vi "set dsf config session.vi"(8 "error in (no error)":errorcluster, 10 "Configuration Session":refnum<class "Configuration Session.lvclass">, 11 "Item Ref in":T1 format="%.0x") -> (0 "error out":errorcluster, 3 "Item Ref out":T1 format="%.0x")   [LabVIEW 2017, in "DSF System Explorer.lvlib"]
uses:
  DSF System Explorer.lvlib
  <vilib>/NI Veristand/Custom Device API/Custom Device Item Ref.ctl
  DSF Core.lvlibp/Classes/Configuration/Configuration Session.lvclass
  <vilib>/NI Veristand/Custom Device API/Custom Device API.lvlib
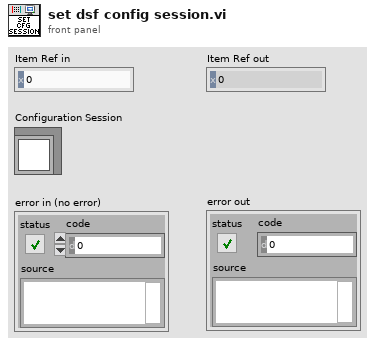
[diagram p1: front panel]
types:
  T1 = typedef "Custom Device API.lvlib/Custom Device Item Ref.ctl" = u64
  T2 = typedef "DSF System Explorer.lvlib/shared data ref.ctl" = refnum<data-value>
  T3 = typedef "DSF System Explorer.lvlib/shared data.ctl" = cluster{"Configuration Session":refnum<class "Configuration Session.lvclass">}
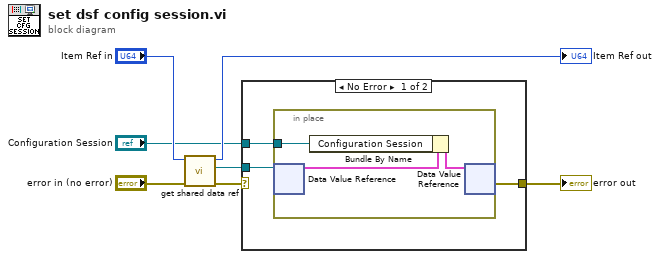
[diagram p0: block diagram]
diagram:
  n1 = call "get shared data ref.vi"("error in (no error)"="error in (no error)", "Node Ptr"="Item Ref in") -> ("error out"=w5:errorcluster, "shared data ref"=w6:T2, "Item Ref out"=→"Item Ref out":T1)  [unwired: 7 in]
  n2 = case shown="No Error" w5 {
    selector: w5 -> [_ w14]
    tunnel: w6 -> [w10 _]
    tunnel: "Configuration Session" -> [w9 _]
    tunnel: [w8 w14] -> w4
    frame No Error {
      n3 = in-place {
        in-place-border: w9 -> [w11]
        n4 = in-place-dvr #1(w10) -> (w12:T3)  [unwired: 1 out]
        n5 = Bundle By Name(cluster=w12, "Configuration Session"=w11) -> (w13:T3)
        n6 = in-place-dvr #1(w13) -> (w8:errorcluster)  [unwired: 1 out]
      }
    }
    frame Error {
    }
  }
  "error out" <- w4
